vi "dgemm - General Matrix-Matrix Product (DBL).vi"(4 "beta":dbl=1.0, 5 "operation B":T1 items=["Direct", "Conjugated & Transposed", "Transposed"], 6 "alpha":dbl=1.0, 7 "operation A":T1 items=["Direct", "Conjugated & Transposed", "Transposed"], 9 "C":T2, 10 "B":T2, 11 "A":T2) -> (0 "error":i32, 3 "dgemm":T2)   [LabVIEW 2020, in "NI_AALBLAS.lvlib"]
doc: "Calculates the product of two general matrices."
uses:
  <vilib>/Analysis/NI_AALBLAS.lvlib
  <vilib>/Analysis/Matrix/Datatypes/RealMatrix.ctl
  <vilib>/Analysis/BLAS.llb/LV_Transpose.ctl
  <vilib>/Analysis/BLAS.llb/Order.ctl
  <vilib>/Analysis/BLAS.llb/Fucntion.ctl
  <vilib>/Analysis/BLAS.llb/BLAS3 Utility(DBL).vi
  <vilib>/Analysis/Matrix/NI_Matrix.lvlib
panel:
  # "dgemm=alpha*op(A)*op(B)+beta*C"
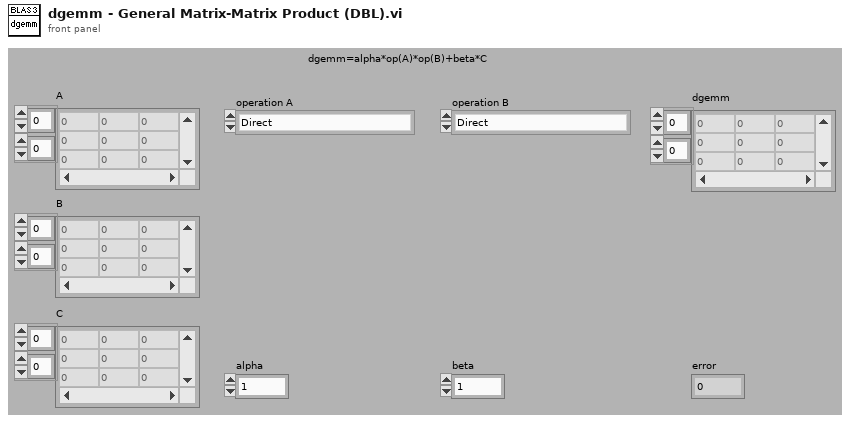
[diagram p1: front panel]
types:
  T1 = typedef "NI_AALBLAS.lvlib/LV_Transpose.ctl" = i32
  T2 = typedef "NI_Matrix.lvlib/RealMatrix.ctl" = dbl[][]
  T3 = typedef "NI_AALBLAS.lvlib/Fucntion.ctl" = u16
  T4 = typedef "NI_AALBLAS.lvlib/Order.ctl" = i32
  T5 = typedef "NI_AALBLAS.lvlib/Operation_Transpose.ctl" = i32
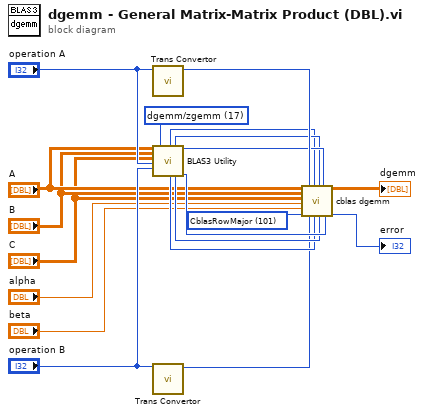
[diagram p0: block diagram]
diagram:
  w1 = T3 17 items=["ddot/zdotu/zdotc", "daxpy/zaxpy", "dnrm2/dznrm2", "dasum/dzasum", "dcopy/zcopy", "dswap/zswap", "drotm", "drot/zdrot", "idamax/izamax", "idamin/izamin", "dgemv/zgemv", "dsymv/zhemv", "dtrmv/ztrmv", "dsyr/zher", "dsyr2/zher2", "dger/zgeru/zgerc", "dtrsv/ztrsv", "dgemm/zgemm", "dsymm/zsymm/zhemm", "dtrmm/ztrmm", "dsyrk/zsyrk/zherk", "dsyr2k/zsyr2k/zher2k", "dtrsm/ztrsm"] ("function")
  w2 = T4 101 items=["CblasRowMajor"=101, "CblasColMajor"=102] ("order")
  n1 = call <vilib>:"Trans Convertor.vi"("operation"="operation A") -> ("trans"=w9:T5)  [unwired: 10 out]
  n2 = call-poly <vilib>:"BLAS3 Utility.vi"("A"="A", "B/X"="B", "C"="C", "operation A"="operation A", "operation B"="operation B", "function"=w1) -> ("lda"=w3:i32, "m"=w15:i32, "ldb/ldx"=w4:i32, "n"=w16:i32, "ldc"=w5:i32, "k"=w17:i32)  [unwired: 8 out]
  n3 = call <vilib>:"Trans Convertor.vi"("operation"="operation B") -> ("trans"=w10:T5)  [unwired: 10 out]
  n4 = call <vilib>:"cblas dgemm.vi"("A"="A", "B"="B", "C"="C", "alpha"="alpha", "beta"="beta", "order"=w2, "transA"=w9, "transB"=w10, "lda"=w3, "m"=w15, "ldb"=w4, "n"=w16, "ldc"=w5, "k"=w17) -> ("dgemm"=→"dgemm":T2, "error"=→"error":i32)  [unwired: 4 out]
